vi "Beta 2.3.1.vi"() -> ()   [LabVIEW 2011]
uses:
  <vilib>/vision/NI_Vision_Development_Module.lvlib
panel:
  in  "Structuring Element":dbl[][](array[numeric])=[[0.0, 1.0, 0.0], [1.0, 1.0, 1.0], [0.0, 1.0, 0.0]]
  in  "Morphology":u16(ring) items=["(none)", "AutoM", "Close", "Dilate", "Erode", "Gradient", "Open", "Thick", "Thin"]
  in  "Generate":bool
  in  "Look for":enum16{"Bright Objects", "Dark Objects"}(ring)
  in  "Method":T1(ring)=enum."Inter-class Variance"
  out "Binary":T2(plugin-control)
  out "Threshold Range":cluster{"Lower value":sgl, "Upper value":sgl}={"Lower value"=128.0, "Upper value"=255.0} {"Upper value" format="%.2f"; "Lower value" format="%.2f"}
  in  "Stop":bool
  in  "Browse":bool
  out "XY Graph":cluster{dbl[], dbl[]}(graph)
  out "Original Image":T2(plugin-control)
  out "Path to Image":path
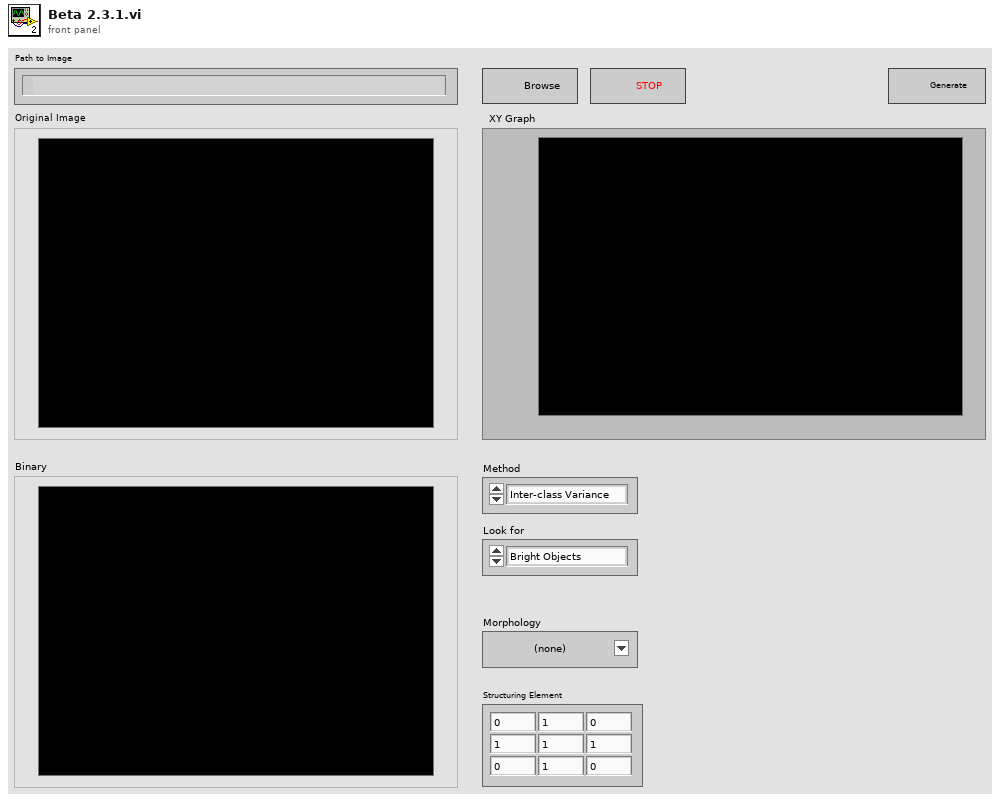
[diagram p1: front panel]
types:
  T1 = enum16{"Clustering", "Entropy", "Metric", "Moments", "Inter-class Variance"}
  T2 = typedef "IMAQ Image.ctl" = refnum<image>
  T3 = typedef "Image Type" = u32
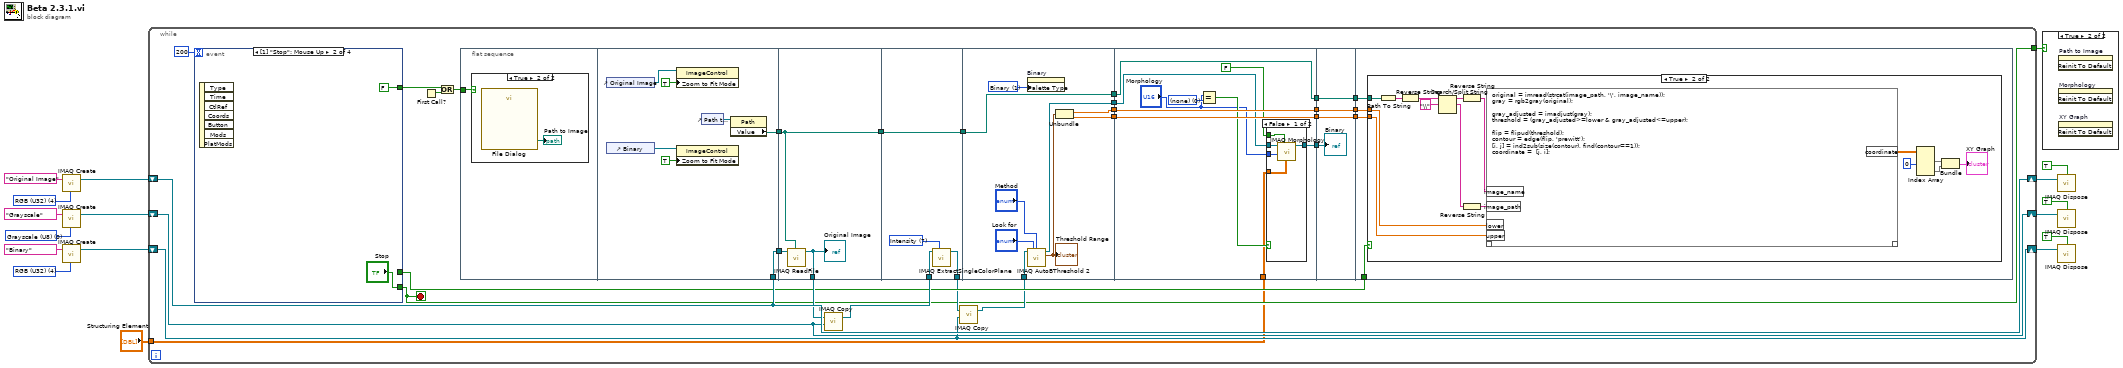
[diagram p0: block diagram]
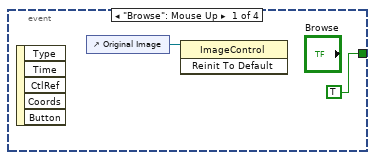
[diagram p3: hidden frame]
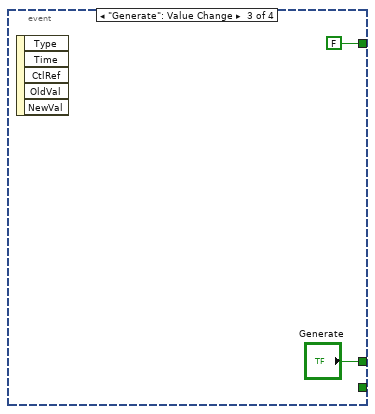
[diagram p4: hidden frame]
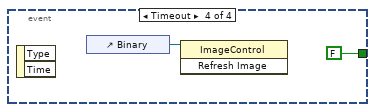
[diagram p5: hidden frame]
diagram:
  w5 = T3 4 items=["Grayscale (U8)", "Grayscale (I16)", "Grayscale (SGL)", "Complex (CSG)", "RGB (U32)", "HSL (U32)", "RGB (U64)", "Grayscale (U16)"] ("Image Type")
  w11 = T3 0 items=["Grayscale (U8)", "Grayscale (I16)", "Grayscale (SGL)", "Complex (CSG)", "RGB (U32)", "HSL (U32)", "RGB (U64)", "Grayscale (U16)"] ("Image Type")
  w16 = T3 4 items=["Grayscale (U8)", "Grayscale (I16)", "Grayscale (SGL)", "Complex (CSG)", "RGB (U32)", "HSL (U32)", "RGB (U64)", "Grayscale (U16)"] ("Image Type")
  n1 = call "IMAQ Create"("Image Name"="Original Image", "Image Type"=w16) -> ("New Image"=w15:T2)  [unwired: 3 in, 1 out]
  n2 = call "IMAQ Create"("Image Name"="Grayscale", "Image Type"=w11) -> ("New Image"=w10:T2)  [unwired: 3 in, 1 out]
  n3 = call "IMAQ Create"("Image Name"="Binary", "Image Type"=w5) -> ("New Image"=w2:T2)  [unwired: 3 in, 1 out]
  n4 = while {
    shift-right: [w41] -> w14
    shift-left: w15 -> [w41]
    tunnel: [w19] -> w13
    shift-right: [w35] -> w8
    shift-left: w10 -> [w35]
    shift-right: [w29] -> w3
    shift-left: w2 -> [w29]
    tunnel: "Structuring Element" -> [w18]
    stop <- w19 stop-if-true
    n5 = event shown="[1] \"Stop\": Mouse Up" {
      selector: _ -> [_ _ _ _]
      dyn-events: _ -> [_ _ _ _]
      timeout: 200 -> [_ _ _ _]
      tunnel: [TRUE FALSE FALSE FALSE] -> w45
      tunnel: [_ "Stop" _ _] -> w19
      tunnel: [_ _ "Generate" _] -> w34
      event "Browse": Mouse Up {
        n6 = event-data() -> ()  [unwired: 1 in, 5 out]
        n7 = control-ref of="Original Image"() -> (w48:refnum<vi>)
        n8 = invoke class="ImageControl" method="Reinit To Default"(reference=w48) -> ()  [unwired: 2 in, 3 out]
      }
      event "Stop": Mouse Up {
        n9 = event-data() -> ()  [unwired: 1 in, 7 out]
      }
      event "Generate": Value Change {
        n10 = event-data() -> ()  [unwired: 1 in, 5 out]
      }
      event Timeout {
        n11 = event-data() -> ()  [unwired: 1 in, 2 out]
        n12 = control-ref of="Binary"() -> (w54:refnum<vi>)
        n13 = invoke class="ImageControl" method="Refresh Image"(reference=w54) -> ()  [unwired: 2 in, 3 out]
      }
    }
    n14 = First Call?() -> (First Call?: T/F=w44:bool)
    n15 = Or(x=w45, y=w44) -> (x .or. y?=w43:bool)
    n16 = flat-sequence {
      tunnel: w43 -> [w55]
      tunnel: [w59] -> w46
      tunnel: [w60] -> w42
      tunnel: w41 -> [w59]
      tunnel: w46 -> [w65]
      tunnel: w42 -> [w66]
      tunnel: [w66] -> w40
      tunnel: [w64] -> w37
      tunnel: w40 -> [w70]
      tunnel: [w70] -> w39
      tunnel: w36 -> [w68]
      tunnel: [w67] -> w30
      tunnel: w39 -> [w79]
      tunnel: [w79] -> w27
      tunnel: [w78] -> w25
      tunnel: [w73] -> w24
      tunnel: [w72] -> w22
      tunnel: w31 -> [w71]
      tunnel: w27 -> [w89]
      tunnel: [w89] -> w26
      tunnel: w25 -> [w86]
      tunnel: w24 -> [w88]
      tunnel: [w88] -> w23
      tunnel: w22 -> [w87]
      tunnel: [w87] -> w21
      tunnel: [w85] -> w20
      tunnel: w18 -> [w80]
      tunnel: w26 -> [w99]
      tunnel: [w99] -> w38
      tunnel: [w98] -> w33
      tunnel: w23 -> [w98]
      tunnel: [w97] -> w32
      tunnel: w21 -> [w97]
      tunnel: w20 -> [w96]
      tunnel: w38 -> [w103]
      tunnel: w34 -> [w102]
      tunnel: w33 -> [w101]
      tunnel: w32 -> [w100]
      frame #0 {
        n17 = case shown="True" w55 {
          frame False {
          }
          frame True {
            n18 = call "File Dialog"() -> ("selected path"=→"Path to Image":path)  [unwired: 12 in, 3 out]
          }
        }
      }
      frame #1 {
        n19 = control-ref of="Original Image"() -> (w63:refnum<vi>)
        n20 = control-ref of="Binary"() -> (w58:refnum<vi>)
        n21 = property class="ImageControl"(reference=w63, "Zoom to Fit Mode"=TRUE) -> ()  [unwired: 1 in, 2 out]
        n22 = property class="ImageControl"(reference=w58, "Zoom to Fit Mode"=TRUE) -> ()  [unwired: 1 in, 2 out]
        n23 = control-ref of="Path to Image"() -> (w61:refnum<vi>)
        n24 = property class="Path"(reference=w61) -> ("Value"=w60:path)  [unwired: 1 in, 2 out]
      }
      frame #2 {
        n25 = call "IMAQ ReadFile"("File Path"=w66, "Image"=w65) -> ("Image Out"=w64:T2)  [unwired: 5 in, 4 out]
        "Original Image" <- w64
      }
      frame #3 {
        w69 = 7 items=["Red", "Green", "Blue", "Hue", "Saturation", "Luminance", "Value", "Intensity"] ("Color Plane")
        n26 = call "IMAQ ExtractSingleColorPlane"("Color Plane"=w69, "Image Src"=w68) -> ("Image Dst Out"=w67:T2)  [unwired: 8 in, 1 out]
      }
      frame #4 {
        w77 = u32 1 items=["Grayscale", "Binary", "Gradient", "Rainbow", "Temperature", "User Defined"] ("Palette")
        n27 = property on="Binary" class="ImageControl"("Palette Type"=w77) -> ()  [unwired: 2 in, 2 out]
        n28 = call "IMAQ AutoBThreshold 2"("Image Src"=w71, "Look For (Bright Objects)"="Look for", "Method (clustering)"="Method") -> ("Image Dst Out"=w78:T2, "Threshold Range Out"=w74:cluster{"Lower value":sgl, "Upper value":sgl})  [unwired: 10 in, 1 out]
        "Threshold Range" <- w74
        n29 = Unbundle(w74) -> ("Lower value"=w73:sgl, "Upper value"=w72:sgl)
      }
      frame #5 {
        w83 = u16 0 items=["(none)"]
        n30 = Equal?(x="Morphology", y=w83) -> (x = y?=w82:bool)
        n31 = case shown="False" w82 {
          tunnel: w86 -> [w91 w95]
          tunnel: [w92 w95] -> w85
          tunnel: FALSE -> [w93 _]
          tunnel: "Morphology" -> [w94 _]
          tunnel: w80 -> [w90 _]
          frame False {
            n32 = call "IMAQ Morphology"("Structuring Element"=w90, "Square/Hexa (Square)"=w93, "Operation"=w94, "Image Src"=w91) -> ("Image Dst Out"=w92:T2)  [unwired: 6 in, 1 out]
          }
          frame True {
          }
        }
      }
      frame #6 {
        "Binary" <- w96
      }
      frame #7 {
        n33 = case shown="True" w102 {
          tunnel: w103 -> [_ w118]
          tunnel: w101 -> [_ w105]
          tunnel: w100 -> [_ w104]
          frame False {
          }
          frame True {
            n34 = Path To String(path=w118) -> (string=w117:string)
            n35 = Reverse String(1:w117) -> (0:w116:string)
            n36 = Search/Split String(string=w116, search string/char (-)="\\") -> (substring before match=w114:string, match + rest of string=w113:string)  [unwired: 1 in, 1 out]
            n37 = Reverse String(1:w114) -> (0:w112:string)
            n38 = Reverse String(1:w113) -> (0:w111:string)
            n39 = script code="original = imread(strcat(image_path, '\\', image_name));\ngray = rgb2gray(original);\n\ngray_adjusted = imadjust(gray);\nthreshold = (gray_adjusted>=lower & gray_adjusted<=upper);\n\nflip = flipud(threshold);\ncontour = edge(flip, 'prewitt');\n[i, j] = ind2sub(size(contour), find(contour==1));\ncoordinate =  [j, i];"("image_name"=w112, "image_path"=w111, "lower"=w105, "upper"=w104) -> ("coordinate"=w110:dbl[][])  [unwired: 1 in, 1 out]
            n40 = Index Array(array=w110, index (col) #1=0 ("disabled index (col)")) -> (element #1=w109:dbl[], element #2=w108:dbl[])  [unwired: 3 in]
            n41 = Bundle(w109, w108) -> (→"XY Graph":cluster{dbl[], dbl[]})  [unwired: 1 in]
          }
        }
      }
    }
    n42 = call "IMAQ Copy"("Image Dst"=w35, "Image Src"=w37) -> ("Image Dst Out"=w36:T2)  [unwired: 4 in, 1 out]
    n43 = call "IMAQ Copy"("Image Dst"=w29, "Image Src"=w30) -> ("Image Dst Out"=w31:T2)  [unwired: 4 in, 1 out]
  }
  n44 = case shown="True" w13 {
    frame False {
    }
    frame True {
      n45 = invoke on="Path to Image" class="Path" method="Reinit To Default"() -> ()  [unwired: 3 in, 3 out]
      n46 = invoke on="Morphology" class="Ring (strict)" method="Reinit To Default"() -> ()  [unwired: 3 in, 3 out]
      n47 = invoke on="XY Graph" class="XYGraph (strict)" method="Reinit To Default"() -> ()  [unwired: 3 in, 3 out]
    }
  }
  n48 = call "IMAQ Dispose"("All Images? (No)"=TRUE, "Image"=w14) -> ()  [unwired: 4 in, 1 out]
  n49 = call "IMAQ Dispose"("All Images? (No)"=TRUE, "Image"=w8) -> ()  [unwired: 4 in, 1 out]
  n50 = call "IMAQ Dispose"("All Images? (No)"=TRUE, "Image"=w3) -> ()  [unwired: 4 in, 1 out]
